vi "test counter.vi"() -> ()   [LabVIEW 2020]
panel:
  out "Counts":i32
  in  "Numeric":i32
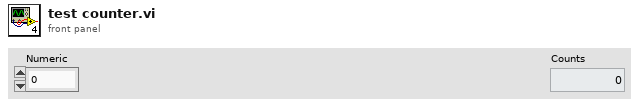
[diagram p1: front panel]
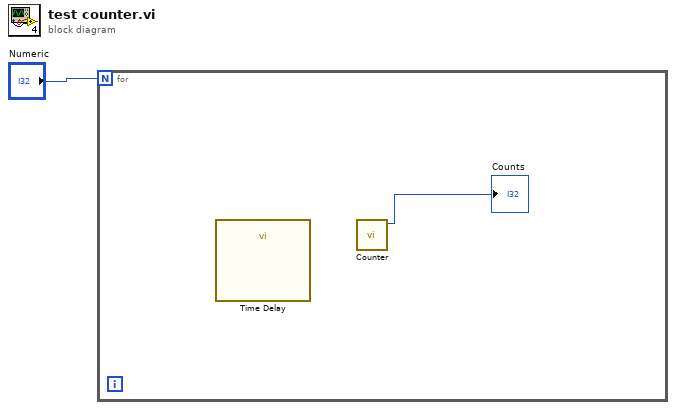
[diagram p0: block diagram]
diagram:
  n1 = for {
    N: "Numeric" -> [_]
    n2 = call "Time Delay"() -> ()  [unwired: 11 in, 1 out]
    n3 = call "Counter.vi"() -> ("counts"=→"Counts":i32)  [unwired: 10 in]
  }
